vi "Main.vi"   [LabVIEW 2021]
uses:
  ABD/ABD/ABD.lvclass
  C:/PPLs/LabVIEW-Composed-Actor-Model-LVCAM/LabVIEW-Composed-Actor-Model-LVCAM/LVCAM/LVCAM/LVCAM/LVCAM.lvclass
  LVCAM/LVCAM/Actor/Actor.lvclass
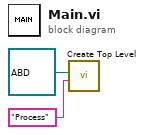
[diagram p0: block diagram]
diagram:
  n1 = call "Create Top Level.vi"("Alias"="Process", "Actor"=refnum<class "ABD.lvclass"> refnum ("Process.lvlib:Process.lvclass")) -> ()  [unwired: 10 in]
